vi "Calculate.vi"(8 "error in (no error)":errorcluster, 9 "Operand 2":dbl, 10 "Operand 1":dbl, 11 "Addition in":refnum<class "Divide.lvclass">) -> (0 "error out":errorcluster, 3 "Addition out":refnum<class "Divide.lvclass">)   [LabVIEW 2013, in "Operators.lvlib" / "Divide.lvclass"]
uses:
  Divide.lvclass
  Divide.lvclass/Divide.ctl
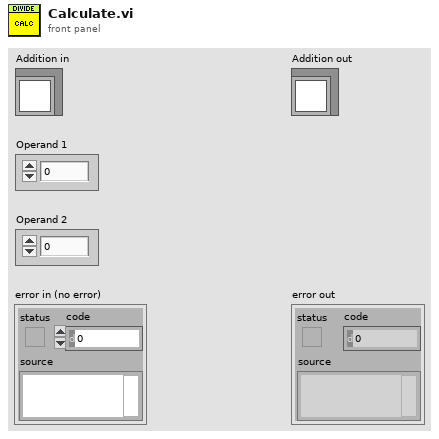
[diagram p1: front panel]
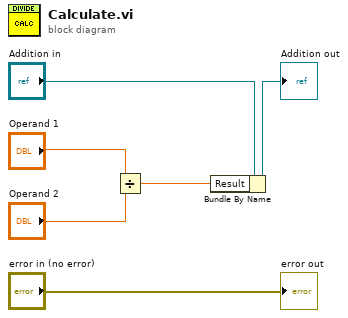
[diagram p0: block diagram]
diagram:
  n1 = Divide(x="Operand 1", y="Operand 2") -> (x/y=w1:dbl)
  n2 = Bundle By Name(cluster="Addition in", "Result"=w1) -> (→"Addition out":refnum<class "Divide.lvclass">)
  "error out" <- "error in (no error)"
